vi "Automatic_spraying_serial_V2.vi"() -> ()   [LabVIEW 2015]
uses:
  <vilib>/Instr/_visa.llb/VISA Configure Serial Port (Instr).vi
panel:
  out "Arduino error report":string
  in  "Tab Control":T1(tab)
  in  "VISA resource name":refnum<visa-resource-name>
  out "error out":errorcluster
  in  "Apply changes":bool
  in  "Pluse set %":dbl(slide) scale=0.0..100.0
  in  "Time limit /s":dbl
  in  "Time limit on":bool
  in  "Upper temp limit /°C":dbl
  in  "Lower temp limit /°C":dbl
  in  "Temprature limit on":bool
  in  "Amplitude set %":dbl(slide) scale=0.0..100.0
  in  "Wait time":dbl
  in  "Number of passes":i8
  in  "Spray type":string(combo)
  in  "Step type":u16(ring) items=["Sixteenth step", "Eighth step", "Quater step", "Half step", "Full step"]
  in  "Heater on/off (on = up)":bool
  in  "Heater temp":i32
  out "Heater on":bool
  in  "stop":bool
  in  "Print":bool
  out "Connected to arduino":bool
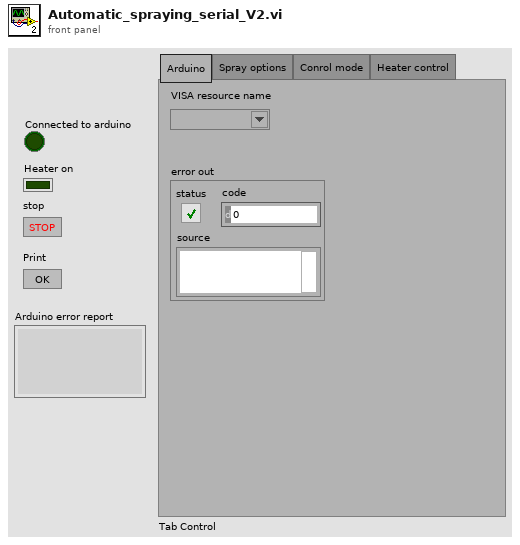
[diagram p1: front panel]
types:
  T1 = enum32{"Arduino", "Spray options", "Conrol mode", "Heater control"}
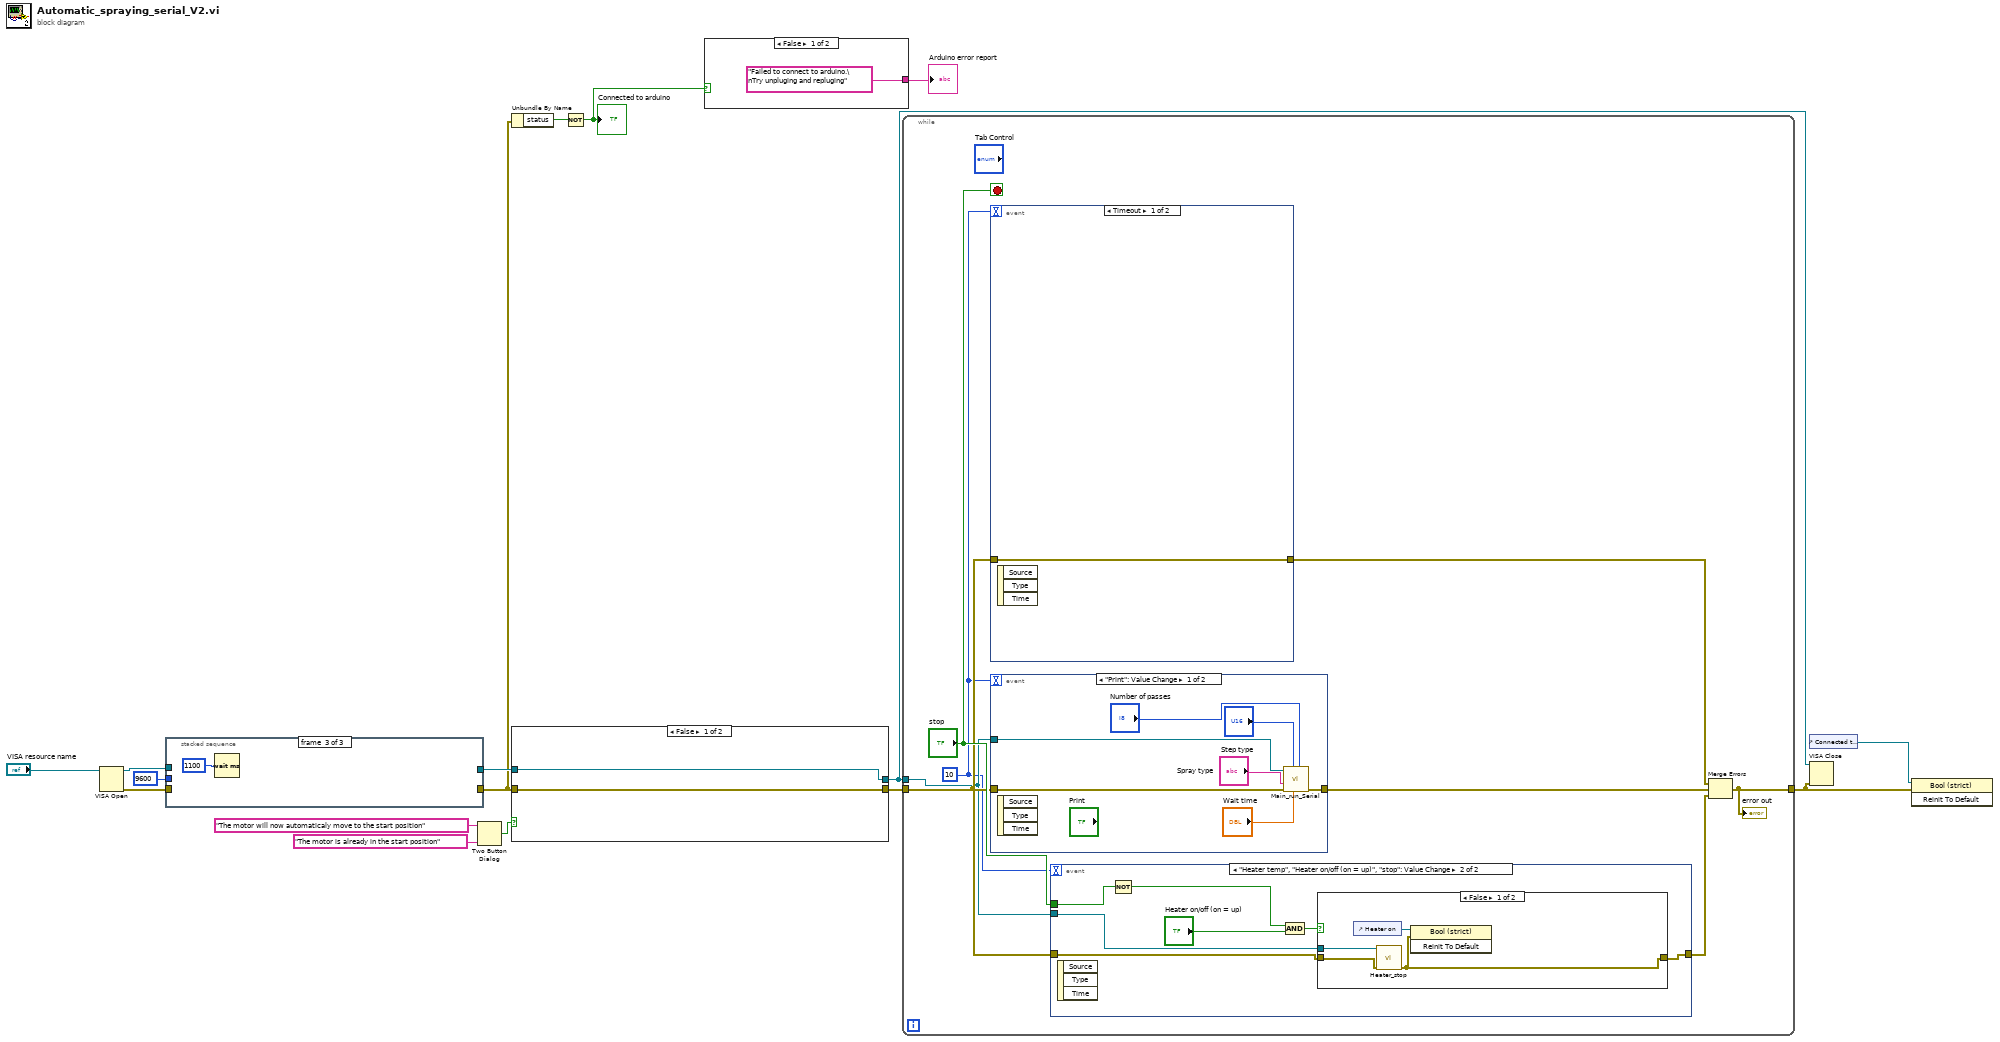
[diagram p0: block diagram]
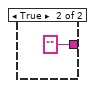
[diagram p2: hidden frame]
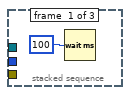
[diagram p3: hidden frame]
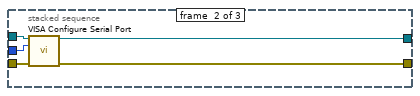
[diagram p4: hidden frame]
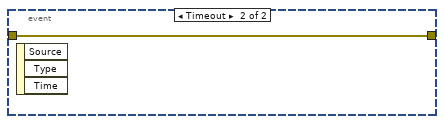
[diagram p5: hidden frame]
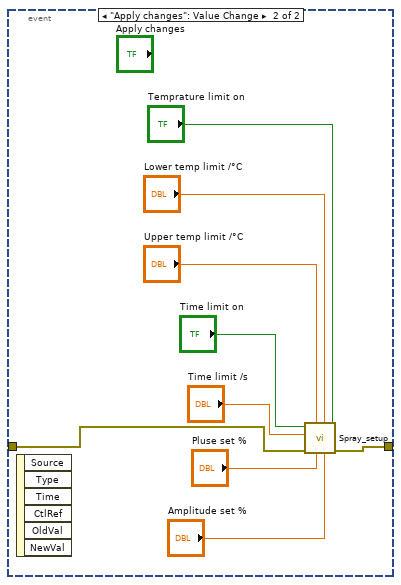
[diagram p6: hidden frame]
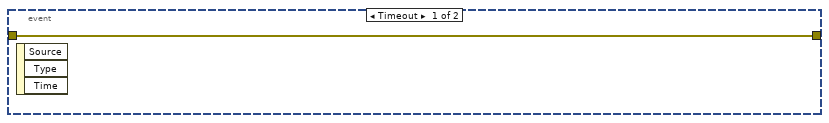
[diagram p7: hidden frame]
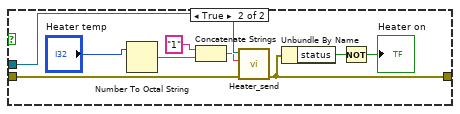
[diagram p8: hidden frame]
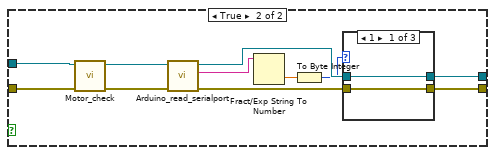
[diagram p9: hidden frame]
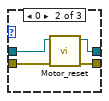
[diagram p10: hidden frame]
diagram:
  n1 = VISA Open(VISA resource name="VISA resource name") -> (VISA resource name=w10:refnum<visa-resource-name>, error out=w9:errorcluster)  [unwired: 4 in]
  n2 = stacked-sequence {
    tunnel: u32 9600 ("baud rate (9600)") -> [_ w22 _]
    tunnel: w10 -> [_ w21 _]
    tunnel: w9 -> [_ w20 _]
    tunnel: [_ w19 _] -> w7
    tunnel: [_ w18 _] -> w6
    frame #0 {
      n3 = Wait (ms)(milliseconds to wait=u32 100) -> ()  [unwired: 1 out]
    }
    frame #1 {
      n4 = call-poly "VISA Configure Serial Port"("VISA resource name"=w21, "baud rate (9600)"=w22, "error in (no error)"=w20) -> ("VISA resource name out"=w19:refnum<visa-resource-name>, "error out"=w18:errorcluster)  [unwired: 11 in]
    }
    frame #2 {
      n5 = Wait (ms)(milliseconds to wait=u32 1100) -> ()  [unwired: 1 out]
    }
  }
  n6 = Two Button Dialog(message="The motor will now automaticaly move to the start position", 1:"The motor is already in the start position" ("F button name (\"Cancel\")")) -> (T button?=w14:bool)  [unwired: 1 in]
  n7 = Unbundle By Name(w6) -> ("status"=w3:bool)
  n8 = case shown="False" w14 {
    tunnel: [w24 w36] -> w13
    tunnel: w7 -> [w25 w35]
    tunnel: w6 -> [w24 w34]
    tunnel: [w25 w29] -> w5
    frame False {
    }
    frame True {
      n9 = call "Motor_check.vi"("error in (no error)"=w34, "VISA resource name"=w35) -> ("error out"=w32:errorcluster, "VISA resource name out"=w33:refnum<visa-resource-name>)  [unwired: 8 in]
      n10 = call "Arduino_read_serialport.vi"("error in (no error)"=w32, "reference"=w33) -> ("error out"=w31:errorcluster, "String"=w28:string, "VISA resource name out"=w30:refnum<visa-resource-name>)  [unwired: 6 in, 1 out]
      n11 = Fract/Exp String To Number(string=w28) -> (number=w27:dbl)  [unwired: 3 in, 1 out]
      n12 = To Byte Integer(number=w27) -> (8bit integer=w26:i8)
      n13 = case shown="1" w26 {
        tunnel: [w38 w40 w43] -> w36
        tunnel: w31 -> [w38 w41 w43]
        tunnel: w30 -> [w37 w42 w44]
        tunnel: [w37 w39 w44] -> w29
        frame 1 {
        }
        frame 0 {
          n14 = call "Motor_reset.vi"("error in (no error)"=w41, "VISA resource name"=w42) -> ("error out"=w40:errorcluster, "VISA resource name out"=w39:refnum<visa-resource-name>)  [unwired: 8 in]
        }
        frame Default {
        }
      }
    }
  }
  n15 = Not(x=w3) -> (.not. x?=w2:bool)
  "Connected to arduino" <- w2
  n16 = case shown="False" w2 {
    tunnel: ["Failed to connect to arduino.\nTry unpluging and repluging" ""] -> w1
    frame False {
    }
    frame True {
    }
  }
  "Arduino error report" <- w1
  n17 = while {
    tunnel: w13 -> [w53]
    tunnel: [w47] -> w4
    tunnel: w5 -> [w50]
    stop <- "stop" stop-if-true
    w48 = 10
    n18 = event shown="[0] Timeout" {
      selector: _ -> [_ _]
      dyn-events: _ -> [_ _]
      timeout: w48 -> [_ _]
      tunnel: [w63 w65] -> w52
      tunnel: w53 -> [w63 w64]
      event Timeout {
        n19 = event-data() -> ()  [unwired: 1 in, 3 out]
      }
      event "Apply changes": Value Change {
        n20 = event-data() -> ()  [unwired: 1 in, 6 out]
        n21 = call "Spray_setup.vi"("Temp limit on"="Temprature limit on", "Amplitude"="Amplitude set %", "Lower temp limit"="Lower temp limit /°C", "Pulse"="Pluse set %", "Upper temp limit"="Upper temp limit /°C", "error in (no error)"=w64, "Time limit"="Time limit /s", "Time limit on"="Time limit on") -> ("error out"=w65:errorcluster)  [unwired: 3 in]
      }
    }
    n22 = event shown="[0] \"Print\": Value Change" {
      selector: _ -> [_ _]
      dyn-events: _ -> [_ _]
      timeout: w48 -> [_ _]
      tunnel: w53 -> [w57 w62]
      tunnel: w50 -> [w59 _]
      tunnel: [w55 w62] -> w49
      event "Print": Value Change {
        n23 = event-data() -> ()  [unwired: 1 in, 3 out]
        n24 = call "Main_run_Serial.vi"("Number of passes"="Number of passes", "Wait time/s"="Wait time", "Step type"="Step type", "error in (no error)"=w57, "Spray Type"="Spray type", "VISA resource name 2"=w59) -> ("error out"=w55:errorcluster)  [unwired: 4 in, 1 out]
      }
      event Timeout {
        n25 = event-data() -> ()  [unwired: 1 in, 3 out]
      }
    }
    n26 = event shown="[1] \"Heater temp\", \"Heater on/off (on = up)\", \"stop\": Value Change" {
      selector: _ -> [_ _]
      dyn-events: _ -> [_ _]
      timeout: w48 -> [_ _]
      tunnel: [w73 w80] -> w51
      tunnel: "stop" -> [_ w77]
      tunnel: w53 -> [w73 w75]
      tunnel: w50 -> [_ w74]
      event Timeout {
        n27 = event-data() -> ()  [unwired: 1 in, 3 out]
      }
      event "Heater temp", "Heater on/off (on = up)", "stop": Value Change {
        n28 = event-data() -> ()  [unwired: 1 in, 3 out]
        n29 = Not(x=w77) -> (.not. x?=w79:bool)
        n30 = And(x=w79, y="Heater on/off (on = up)") -> (x .and. y?=w78:bool)
        n31 = case shown="False" w78 {
          tunnel: [w81 w85] -> w80
          tunnel: w75 -> [w83 w87]
          tunnel: w74 -> [w82 w88]
          frame False {
            n32 = control-ref of="Heater on"() -> (w84:refnum<vi>)
            n33 = call "Heater_stop.vi"("error in (no error)"=w83, "VISA resource name"=w82) -> ("error out"=w81:errorcluster)  [unwired: 8 in, 1 out]
            n34 = invoke on="Invoke Node" class="Bool (strict)" method="Reinit To Default"(reference=w84, error in=w81) -> ()  [unwired: 1 in, 3 out]
          }
          frame True {
            n35 = Number To Octal String(2:"Heater temp") -> (0:w89:string)  [unwired: 1 in]
            n36 = Concatenate Strings("1", w89) -> (w86:string)
            n37 = call "Heater_send.vi"("error in (no error)"=w87, "String"=w86, "VISA resource name"=w88) -> ("error out"=w85:errorcluster)  [unwired: 7 in, 1 out]
            n38 = Unbundle By Name(w85) -> ("status"=w92:bool)
            n39 = Not(x=w92) -> (.not. x?=→"Heater on":bool)
          }
        }
      }
    }
    n40 = Merge Errors(w52, w49, w51) -> (w47:errorcluster)
    "error out" <- w47
  }
  n41 = control-ref of="Connected to arduino"() -> (w12:refnum<vi>)
  n42 = VISA Close(VISA resource name=w5, error in (no error)=w4) -> ()  [unwired: 1 out]
  n43 = invoke on="Invoke Node" class="Bool (strict)" method="Reinit To Default"(reference=w12, error in=w4) -> ()  [unwired: 1 in, 3 out]
